vi "Initialize Edit Mode.vi"(8 "error in (no error)":errorcluster, 11 "Numeric Data Type in":refnum<class "Numeric Data Type.lvclass">) -> (0 "error out":errorcluster, 3 "Numeric Data Type (dup)":refnum<class "Numeric Data Type.lvclass">)   [LabVIEW 2018, in "Numeric Data Type.lvclass"]
uses:
  Numeric Data Type.lvclass
  Numeric Data Type.lvclass/Numeric Data Type.ctl
  Reference Editing Mode.vi
  Reference Default-Advanced Tab.vi
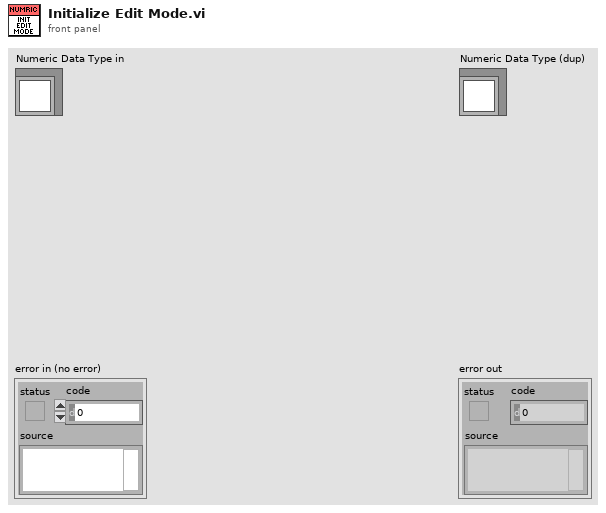
[diagram p1: front panel]
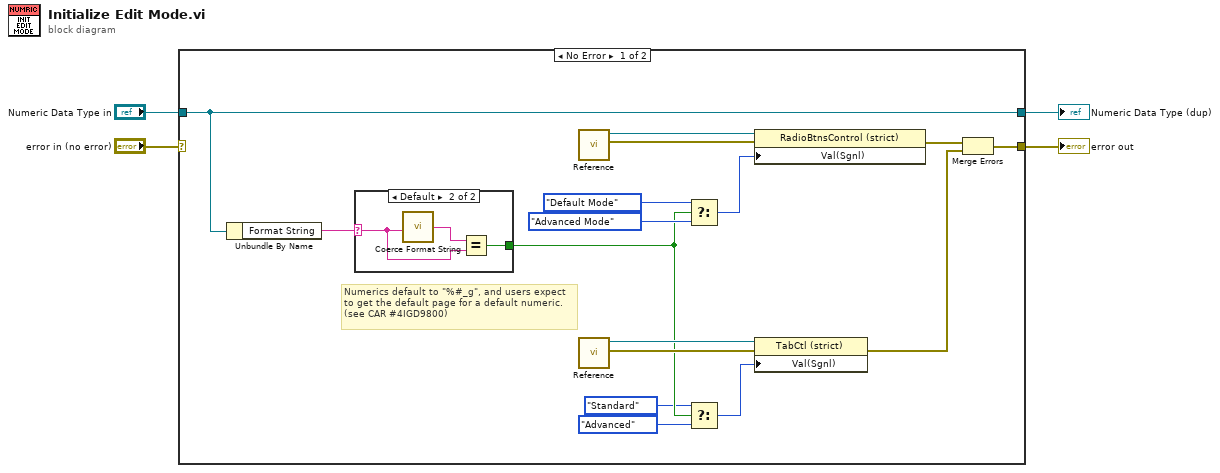
[diagram p0: block diagram]
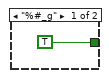
[diagram p2: hidden frame]
diagram:
  n1 = case shown="No Error" "error in (no error)" {
    selector: "error in (no error)" -> [_ w26]
    tunnel: [w6 w26] -> w3
    tunnel: [w20 w25] -> w1
    tunnel: "Numeric Data Type in" -> [w20 w25]
    frame No Error {
      # "Numerics default to \"%#_g\", and users expect to get the default page for a default numeric.\n(see CAR #4IGD9800)"
      n2 = Unbundle By Name(w20) -> ("Format String"=w19:string)
      n3 = case shown="Default" w19 {
        selector: w19 -> [_ w23]
        tunnel: [TRUE w24] -> w10
        frame "%#_g" {
        }
        frame Default {
          n4 = call "Coerce Format String.vi"("Format String"=w23) -> ("Coerced String"=w22:string)
          n5 = Equal?(x=w22, y=w23) -> (x = y?=w24:bool)
        }
      }
      n6 = call-poly "Reference.vi"() -> ("error out"=w13:errorcluster, "Editing Mode"=w14:refnum<vi>)  [unwired: 10 in]
      n7 = call-poly "Reference.vi"() -> ("error out"=w11:errorcluster, "Default/Advanced Tab"=w12:refnum<vi>)  [unwired: 10 in]
      n8 = Select(t=enum32{"Default Mode", "Advanced Mode"}."Default Mode" ("Value (Signaling)"), s=w10, f=enum32{"Default Mode", "Advanced Mode"}."Advanced Mode" ("Value (Signaling)")) -> (s? t:f=w16:enum32{"Default Mode", "Advanced Mode"})
      n9 = Select(t=enum32{"Standard", "Advanced"}."Standard" ("Value (Signaling)"), s=w10, f=enum32{"Standard", "Advanced"}."Advanced" ("Value (Signaling)")) -> (s? t:f=w7:enum32{"Standard", "Advanced"})
      n10 = property class="RadioBtnsControl (strict)"(reference=w14, error in=w13, "Val(Sgnl)"=w16) -> (error out=w15:errorcluster)  [unwired: 1 out]
      n11 = property class="TabCtl (strict)"(reference=w12, error in=w11, "Val(Sgnl)"=w7) -> (error out=w5:errorcluster)  [unwired: 1 out]
      n12 = Merge Errors(w15, w5) -> (w6:errorcluster)
    }
    frame Error {
    }
  }
  "error out" <- w3
  "Numeric Data Type (dup)" <- w1
